vi "AIT 429 Main Page.vi"(8 "error in (no error)":errorcluster, 11 "Node Ptr":T2 format="%.0x") -> (0 "error out":errorcluster)   [LabVIEW 2012, in "AIT 429 System Explorer.lvlib"]
uses:
  AIT 429 System Explorer.lvlib
  <vilib>/NI Veristand/Custom Device API/Custom Device Item Ref.ctl
  Shared/Controls and Global/Specify module by.ctl
  Shared/Controls and Global/Global.vi
  <vilib>/NI Veristand/Custom Device API/Get Item Property (Boolean).vi
  <vilib>/NI Veristand/Custom Device API/Get Item Property (Path).vi
  <vilib>/NI Veristand/Custom Device API/Get Item Property (Variant).vi
  <vilib>/NI Veristand/Custom Device API/Get Item Property (U16).vi
  <vilib>/NI Veristand/Custom Device API/Get Item Property (String).vi
  <vilib>/NI Veristand/Custom Device API/Set Item Property (Variant).vi
  <vilib>/NI Veristand/Custom Device API/Set Item Property (String).vi
  <vilib>/NI Veristand/Custom Device API/Set Item Property (U16).vi
  <vilib>/NI Veristand/Custom Device API/Custom Device API.lvlib
  Shared/ARINC 429 Shared.lvlib
  <vilib>/NI Veristand/Custom Device API/Set Item Property (Boolean).vi
panel:
  in  "Specify module by":T1
  out "Version":string
  in  "ScheduledSDI?":bool
  in  "RefreshDB":bool
  in  "Warning text":string="WARNING: The database has changed since import. If you attempt to run this system definition an error may occur. Consider refreshing the database import."
  out "Warn Icon":bool
  out "Database File":path
  in  "Module":u64
  in  "Header":cluster{"Section Name":string}={"Section Name"="ARINC 429 - AIT -  Custom Device"}
  in  "Description":string
  in  "Name":string
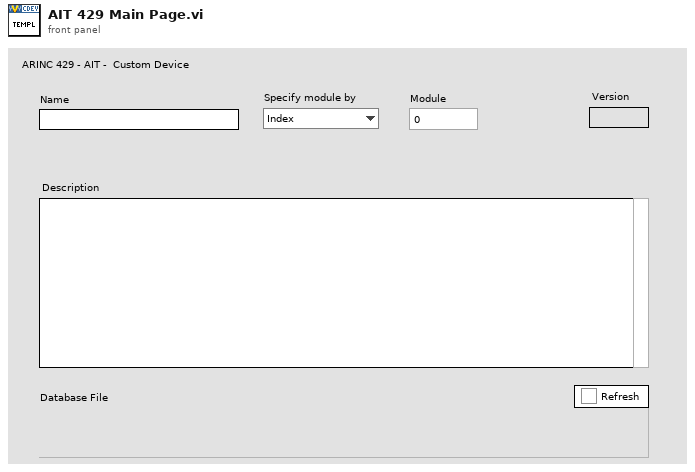
[diagram p1: front panel]
types:
  T1 = typedef "ARINC 429 Shared.lvlib/Specify module by.ctl" = enum16{"Index", "SlotID", "Serial number"}
  T2 = typedef "Custom Device API.lvlib/Custom Device Item Ref.ctl" = u64
  T3 = typedef "Custom Device API.lvlib/Custom Device Item Info.ctl" = cluster{"Name":string, "Is Channel":bool, "GUID":string, "Is Waveform":bool}
  T4 = typedef "Custom Device API.lvlib/Custom Device Commands.ctl" = enum16{"Default", "Item renamed", "Shutdown", "Dynamic button pressed"}
  T5 = typedef "AIT 429 System Explorer.lvlib/Refresh Match Settings.ctl" = cluster{"Ch by name?":bool, "Lbl by name?":bool}
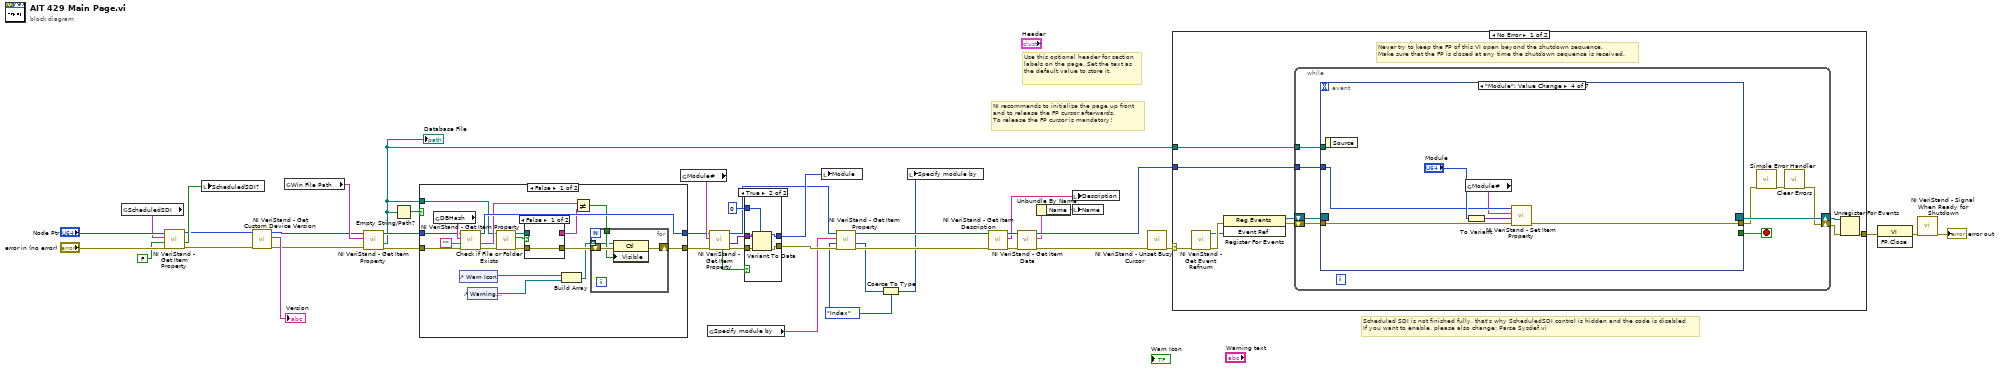
[diagram p0: block diagram]
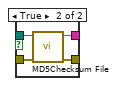
[diagram p2: hidden frame]
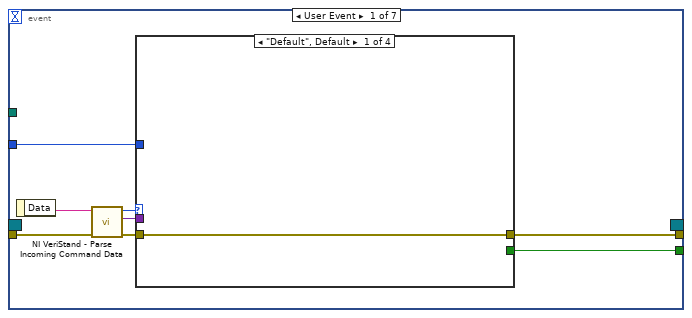
[diagram p5: hidden frame]
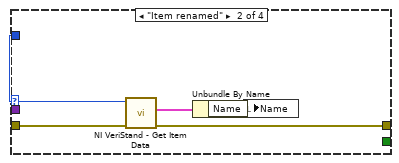
[diagram p6: hidden frame]
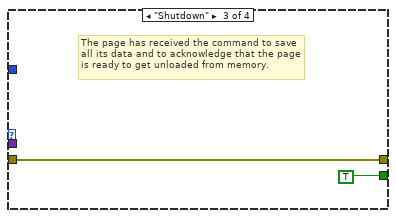
[diagram p7: hidden frame]
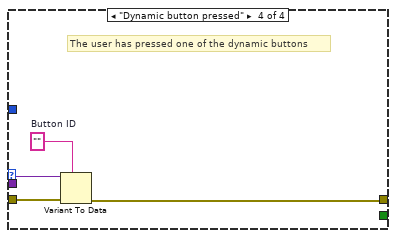
[diagram p8: hidden frame]
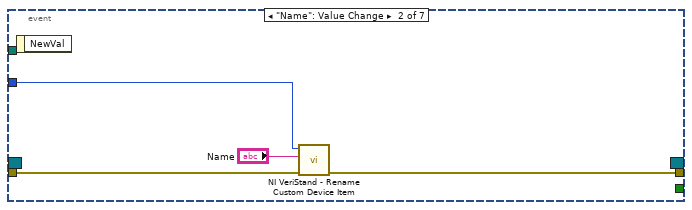
[diagram p9: hidden frame]
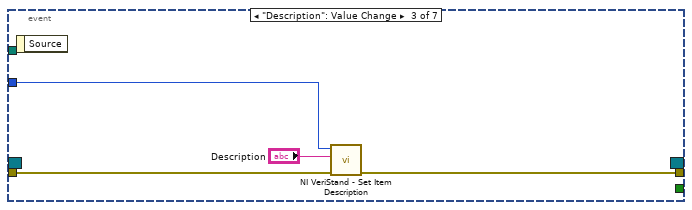
[diagram p10: hidden frame]
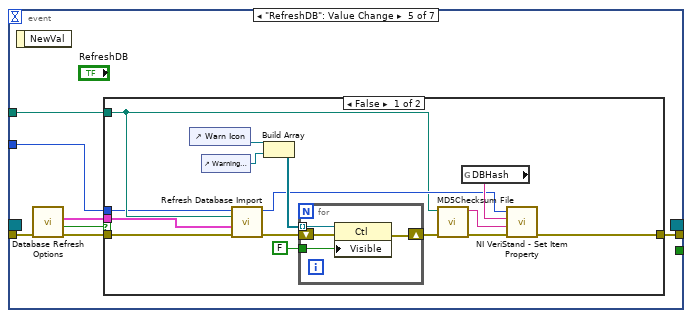
[diagram p11: hidden frame]
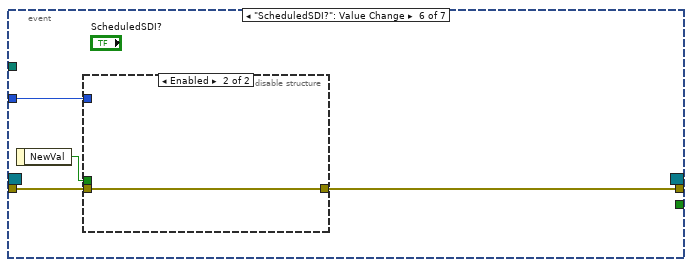
[diagram p13: hidden frame]
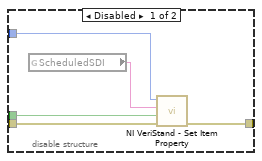
[diagram p14: hidden frame]
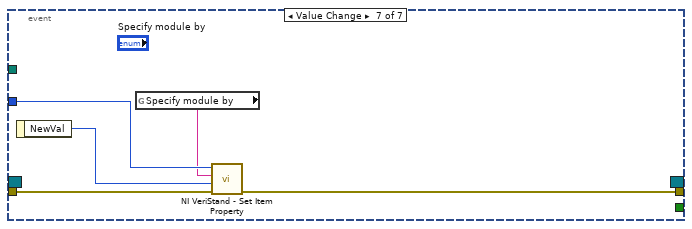
[diagram p15: hidden frame]
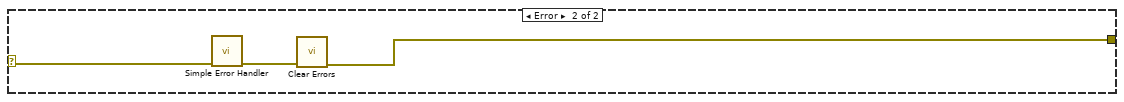
[diagram p16: hidden frame]
diagram:
  w2 = Specify_module_by."Index" ("Specify module by")
  # "Scheduled SDI is not finished fully, that's why ScheduledSDI control is hidden and the code is disabled\nIf you want to enable, please also change: Parse Sysdef.vi"
  # "Use this optional header for section labels on the page. Set the text as the default value to store it."
  # "NI recommends to initialize the page up front\nand to release the FP cursor afterwards.\nTo release the FP cursor is mandatory!"
  n1 = global read "Global.vi" "ScheduledSDI"() -> (w15:string)
  n2 = call-poly <vilib>:"NI VeriStand - Get Item Property.vi"("error in (no error)"="error in (no error)", "Default Value"=FALSE, "Property Name"=w15, "Item Ref in"="Node Ptr") -> ("error out"=w16:errorcluster, "Value"=w13:bool, "Item Ref out"=w12:T2)  [unwired: 4 in, 1 out]
  n3 = local write "ScheduledSDI?"(w13) -> ()
  n4 = call <vilib>:"NI VeriStand - Get Custom Device Version.vi"("error in (no error)"=w16, "Device Ref in"=w12) -> ("error out"=w9:errorcluster, "Value"=→"Version":string, "Device Ref out"=w10:T2)  [unwired: 7 in]
  n5 = global read "Global.vi" "Win File Path"() -> (w31:string)
  n6 = call-poly <vilib>:"NI VeriStand - Get Item Property.vi"("error in (no error)"=w9, "Property Name"=w31, "Item Ref in"=w10) -> ("error out"=w23:errorcluster, "Value"=w19:path, "Item Ref out"=w20:T2)  [unwired: 5 in, 1 out]
  "Database File" <- w19
  n7 = Empty String/Path?(string/path=w19) -> (empty?=w24:bool)
  n8 = case shown="False" w24 {
    tunnel: w23 -> [w57 w71]
    tunnel: [w48 w71] -> w22
    tunnel: [w56 w70] -> w21
    tunnel: w20 -> [w58 w70]
    tunnel: w19 -> [w44 _]
    frame False {
      n9 = global read "Global.vi" "DBHash"() -> (w59:string)
      n10 = control-ref of="Warn Icon"() -> (w50:refnum<vi>)
      n11 = call-poly <vilib>:"NI VeriStand - Get Item Property.vi"("error in (no error)"=w57, "Default Value"="", "Property Name"=w59, "Item Ref in"=w58) -> ("error out"=w45:errorcluster, "Value"=w54:string, "Item Ref out"=w56:T2)  [unwired: 4 in, 1 out]
      n12 = control-ref of="Warning text"() -> (w51:refnum<vi>)
      n13 = call <vilib>:"Check if File or Folder Exists.vi"("error in (no error)"=w45, "path"=w44) -> ("error out"=w47:errorcluster, "file or folder exists?"=w43:bool, "dup path"=w46:path)  [unwired: 7 in]
      n14 = case shown="False" w43 {
        tunnel: [_ w65] -> w55
        tunnel: [w61 w64] -> w53
        tunnel: w47 -> [w61 w63]
        tunnel: w46 -> [_ w62]
        frame False {
        }
        frame True {
          n15 = call <vilib>:"MD5Checksum File.vi"("error in (no error)"=w63, "Path"=w62) -> ("error out"=w64:errorcluster, "MD5 message-digest"=w65:string)  [unwired: 8 in]
        }
      }
      n16 = Build Array(w50, w51) -> (w49:refnum<vi>[])
      n17 = Not Equal?(x=w54, y=w55) -> (x != y?=w52:bool)
      n18 = for {
        shift-right: [w68] -> w48
        shift-left: w53 -> [w69]
        tunnel: w52 -> [w67]
        tunnel: w49 -> [w66] mode=indexing
        n19 = property class="Ctl"(reference=w66, error in=w69, "Visible"=w67) -> (error out=w68:errorcluster)  [unwired: 1 out]
      }
    }
    frame True {
    }
  }
  n20 = global read "Global.vi" "Module#"() -> (w30:string)
  n21 = global read "Global.vi" "Specify module by"() -> (w5:string)
  n22 = call-poly <vilib>:"NI VeriStand - Get Item Property.vi"("error in (no error)"=w22, "Property Name"=w30, "Item Ref in"=w21) -> ("error out"=w29:errorcluster, "Value"=w25:variant, "Item Ref out"=w7:T2, "Found?"=w3:bool)  [unwired: 5 in]
  n23 = case shown="True" w3 {
    tunnel: w29 -> [w72 w78]
    tunnel: [w72 w77] -> w28
    tunnel: u64 0 ("Board Serial #") -> [w73 w76]
    tunnel: [w73 w75] -> w26
    tunnel: w25 -> [_ w74]
    frame False {
    }
    frame True {
      n24 = Variant To Data(error in=w78, type=w76, Variant=w74) -> (data=w75:u64, error out=w77:errorcluster)
    }
  }
  n25 = local write "Module"(w26) -> ()
  n26 = call-poly <vilib>:"NI VeriStand - Get Item Property.vi"("error in (no error)"=w28, "Default Value"=w2, "Property Name"=w5, "Item Ref in"=w7) -> ("error out"=w8:errorcluster, "Value"=w4:u16, "Item Ref out"=w6:T2)  [unwired: 4 in, 1 out]
  n27 = Coerce To Type(0:w4, 1:w2) -> (2:w1:T1)
  n28 = local write "Specify module by"(w1) -> ()
  n29 = call <vilib>:"NI VeriStand - Get Item Description.vi"("error in (no error)"=w8, "Item Ref in"=w6) -> ("error out"=w34:errorcluster, "Description"=w35:string, "Item Ref out"=w36:T2)  [unwired: 7 out]
  n30 = call <vilib>:"NI VeriStand - Get Item Data.vi"("error in (no error)"=w34, "Item Ref in"=w36) -> ("error out"=w39:errorcluster, "Item Info"=w33:T3, "Item Ref out"=w37:T2)  [unwired: 7 out]
  n31 = Unbundle By Name(w33) -> ("Name"=w32:string)
  n32 = local write "Description"(w35) -> ()
  n33 = local write "Name"(w32) -> ()
  n34 = call <vilib>:"NI VeriStand - Unset Busy Cursor.vi"("error in (no error)"=w39) -> ("error out"=w38:errorcluster)  [unwired: 10 out]
  n35 = case shown="No Error" w38 {
    selector: w38 -> [w80 w176]
    tunnel: [w85 w174] -> w42
    tunnel: w37 -> [w81 _]
    tunnel: w19 -> [w79 _]
    frame No Error {
      # "Never try to keep the FP of this VI open beyond the shutdown sequence.\nMake sure that the FP is closed at any time the shutdown sequence is received."
      n36 = call <vilib>:"NI VeriStand - Get Event Refnum.vi"("error in (no error)"=w80) -> ("error out"=w88:errorcluster, "Event Ref"=w84:refnum<user-event>)  [unwired: 9 out]
      n37 = register-events(error in=w88, w84) -> (reference out=w82:refnum<event-registration>, error out=w83:errorcluster)  [unwired: 1 in]
      n38 = while {
        tunnel: w81 -> [w93]
        shift-right: [w90] -> w86
        shift-left: w83 -> [w96]
        shift-right: [w97] -> w87
        shift-left: w82 -> [w95]
        tunnel: w79 -> [w89]
        stop <- w94 stop-if-true
        n39 = event shown="[3] \"Module\": Value Change" {
          selector: w95 -> [_ _ _ _ _ _ _]
          dyn-events: [_ _ _ _ _ _ _] -> w97
          timeout: _ -> [_ _ _ _ _ _ _]
          tunnel: w96 -> [w105 w121 w124 w131 w133 w162 w173]
          tunnel: [w101 _ _ _ _ _ _] -> w94
          tunnel: [w100 w120 w123 w130 w132 w159 w169] -> w92
          tunnel: w93 -> [w99 w119 w125 w127 w137 w161 w172]
          tunnel: w89 -> [_ _ _ _ w138 _ _]
          event User Event {
            n40 = event-data() -> ("Data"=w104:string)  [unwired: 1 out]
            n41 = call <vilib>:"NI VeriStand - Parse Incoming Command Data.vi"("error in (no error)"=w105, "Incoming data"=w104) -> ("error out"=w103:errorcluster, "Outgoing data"=w98:variant, "Action"=w102:T4)  [unwired: 7 out]
            n42 = case shown="\"Default\", Default" w102 {
              tunnel: w103 -> [w106 w111 w112 w117]
              tunnel: [_ _ TRUE _] -> w101
              tunnel: [w106 w108 w112 w114] -> w100
              tunnel: w99 -> [_ w110 _ _]
              tunnel: w98 -> [_ _ _ w116]
              frame "Default", Default {
              }
              frame "Item renamed" {
                n43 = call <vilib>:"NI VeriStand - Get Item Data.vi"("error in (no error)"=w111, "Item Ref in"=w110) -> ("error out"=w108:errorcluster, "Item Info"=w109:T3)  [unwired: 8 out]
                n44 = Unbundle By Name(w109) -> ("Name"=w107:string)
                n45 = local write "Name"(w107) -> ()
              }
              frame "Shutdown" {
                # "The page has received the command to save all its data and to acknowledge that the page is ready to get unloaded from memory."
              }
              frame "Dynamic button pressed" {
                w115 = ""  # Button ID
                # "The user has pressed one of the dynamic buttons"
                n46 = Variant To Data(error in=w117, type=w115, Variant=w116) -> (error out=w114:errorcluster)  [unwired: 1 out]
              }
            }
          }
          event "Name": Value Change {
            n47 = event-data() -> ()  [unwired: 2 out]
            n48 = call <vilib>:"NI VeriStand - Rename Custom Device Item.vi"("error in (no error)"=w121, "New Name"="Name", "Item Ref in"=w119) -> ("error out"=w120:errorcluster)  [unwired: 1 in, 7 out]
          }
          event "Description": Value Change {
            n49 = event-data() -> ()  [unwired: 2 out]
            n50 = call <vilib>:"NI VeriStand - Set Item Description.vi"("error in (no error)"=w124, "Description"="Description", "Item Ref in"=w125) -> ("error out"=w123:errorcluster)  [unwired: 8 out]
          }
          event "Module": Value Change {
            n51 = event-data() -> ()  [unwired: 2 out]
            n52 = global read "Global.vi" "Module#"() -> (w126:string)
            n53 = To Variant(anything="Module") -> (Variant=w128:variant)
            n54 = call-poly <vilib>:"NI VeriStand - Set Item Property.vi"("error in (no error)"=w131, "Value"=w128, "Property Name"=w126, "Item Ref in"=w127) -> ("error out"=w130:errorcluster)  [unwired: 5 in, 2 out]
          }
          event "RefreshDB": Value Change {
            n55 = event-data() -> ()  [unwired: 2 out]
            n56 = call "Database Refresh Options.vi"("error in (no error)"=w133) -> ("error out"=w136:errorcluster, "Cancelled?"=w135:bool, "Refresh Settings"=w134:T5)  [unwired: 8 in]
            n57 = case shown="False" w135 {
              tunnel: [w140 w158] -> w132
              tunnel: w136 -> [w139 w158]
              tunnel: w138 -> [w143 _]
              tunnel: w137 -> [w142 _]
              tunnel: w134 -> [w141 _]
              frame False {
                n58 = control-ref of="Warn Icon"() -> (w149:refnum<vi>)
                n59 = control-ref of="Warning text"() -> (w150:refnum<vi>)
                n60 = call "Refresh Database Import.vi"("error in (no error)"=w139, "Match settings"=w141, "DB"=w143, "Item Ref in"=w142) -> ("error out"=w145:errorcluster, "Item Ref dup"=w144:T2)  [unwired: 5 in, 1 out]
                n61 = Build Array(w149, w150) -> (w147:refnum<vi>[])
                n62 = for {
                  shift-right: [w156] -> w148
                  shift-left: w145 -> [w157]
                  tunnel: w147 -> [w155] mode=indexing
                  tunnel: FALSE ("Visible") -> [w154]
                  n63 = property class="Ctl"(reference=w155, error in=w157, "Visible"=w154) -> (error out=w156:errorcluster)  [unwired: 1 out]
                }
                n64 = call <vilib>:"MD5Checksum File.vi"("error in (no error)"=w148, "Path"=w143) -> ("error out"=w153:errorcluster, "MD5 message-digest"=w152:string)  [unwired: 8 in]
                n65 = global read "Global.vi" "DBHash"() -> (w151:string)
                n66 = call-poly <vilib>:"NI VeriStand - Set Item Property.vi"("error in (no error)"=w153, "Value"=w152, "Property Name"=w151, "Item Ref in"=w144) -> ("error out"=w140:errorcluster)  [unwired: 5 in, 2 out]
              }
              frame True {
              }
            }
          }
          event "ScheduledSDI?": Value Change {
            n67 = event-data() -> ("NewVal"=w160:bool)  [unwired: 1 out]
            n68 = disable-structure shown="Enabled" {
              disable-tunnel: w162 -> [w167 w168]
              disable-tunnel: w161 -> [w166 _]
              disable-tunnel: w160 -> [w165 _]
              disable-tunnel: [w164 w168] -> w159
              frame Disabled {
                n69 = global read "Global.vi" "ScheduledSDI"() -> (w163:string)
                n70 = call-poly <vilib>:"NI VeriStand - Set Item Property.vi"("error in (no error)"=w167, "Value"=w165, "Property Name"=w163, "Item Ref in"=w166) -> ("error out"=w164:errorcluster)  [unwired: 5 in, 2 out]
              }
              frame Enabled {
              }
            }
          }
          event Value Change {
            n71 = event-data() -> ("NewVal"=w171:T1)  [unwired: 1 out]
            n72 = global read "Global.vi" "Specify module by"() -> (w170:string)
            n73 = call-poly <vilib>:"NI VeriStand - Set Item Property.vi"("error in (no error)"=w173, "Value"=w171, "Property Name"=w170, "Item Ref in"=w172) -> ("error out"=w169:errorcluster)  [unwired: 5 in, 2 out]
          }
        }
        n74 = call <vilib>:"Simple Error Handler.vi"("error in (no error)"=w92) -> ("error out"=w91:errorcluster)  [unwired: 1 in, 7 out]
        n75 = call <vilib>:"Clear Errors.vi"("error in (no error)"=w91) -> ("error out"=w90:errorcluster)  [unwired: 6 out]
      }
      n76 = Unregister For Events(event registration refnum=w87, error in=w86) -> (error out=w85:errorcluster)
    }
    frame Error {
      n77 = call <vilib>:"Simple Error Handler.vi"("error in (no error)"=w176) -> ("error out"=w175:errorcluster)  [unwired: 1 in, 7 out]
      n78 = call <vilib>:"Clear Errors.vi"("error in (no error)"=w175) -> ("error out"=w174:errorcluster)  [unwired: 6 out]
    }
  }
  n79 = invoke class="VI" method="FP.Close"(error in=w42) -> (error out=w41:errorcluster)  [unwired: 2 in, 2 out]
  n80 = call <vilib>:"NI VeriStand - Signal When Ready for Shutdown.vi"("error in (no error)"=w41) -> ("error out"=→"error out":errorcluster)  [unwired: 10 out]
